vi "NotifyWithDataOverride.vi"(8 "error in (no error)":errorcluster, 11 "TCP Com in":refnum<class "TCP Com.lvclass">) -> (0 "error out":errorcluster, 2 "Data out":refnum<class "Data.lvclass">, 3 "TCP Com out":refnum<class "TCP Com.lvclass">)   [LabVIEW 2023, in "TCP Com.lvclass"]
uses:
  TCP Com.lvclass
  C:/Users/santharu.subramanian/Desktop/LOA New/Documents/LV New Assignments/Sender-Receiver/Classes/Communication/Communication.lvclass
  Data/Data.lvclass
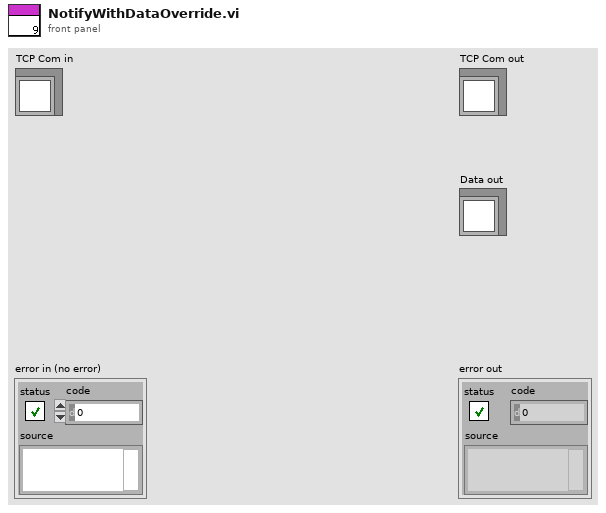
[diagram p1: front panel]
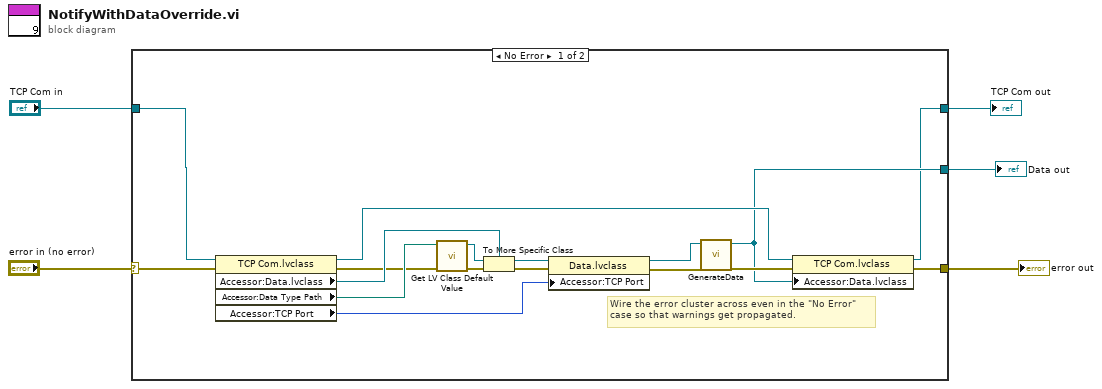
[diagram p0: block diagram]
diagram:
  n1 = case shown="No Error" "error in (no error)" {
    selector: "error in (no error)" -> [w7 w24]
    tunnel: [w6 w24] -> w4
    tunnel: [w8 w23] -> w2
    tunnel: "TCP Com in" -> [w10 w23]
    tunnel: [w9 _] -> w1
    frame No Error {
      # "Wire the error cluster across even in the \"No Error\"\ncase so that warnings get propagated."
      n2 = property class="TCP Com.lvclass"(reference=w10, error in=w7) -> (reference out=w16:refnum<class "TCP Com.lvclass">, error out=w17:errorcluster, "Accessor:Data.lvclass"=w18:refnum<class "Data.lvclass">, "Accessor:Data Type Path"=w19:path, "Accessor:TCP Port"=w11:u16)
      n3 = call <vilib>:"Get LV Class Default Value.vi"("error in (no error)"=w17, "class path"=w19) -> ("error out"=w22:errorcluster, "object"=w21:refnum<class>)  [unwired: 8 in]
      n4 = To More Specific Class(target class=w18, reference=w21, error in=w22) -> (specific class reference=w20:refnum<class "Data.lvclass">, error out=w13:errorcluster)
      n5 = property class="Data.lvclass"(reference=w20, error in=w13, "Accessor:TCP Port"=w11) -> (reference out=w14:refnum<class "Data.lvclass">, error out=w12:errorcluster)
      n6 = call-dynamic "GenerateData.vi"("error in (no error)"=w12, "Data in"=w14) -> ("error out"=w15:errorcluster, "Data out"=w9:refnum<class "Data.lvclass">)  [unwired: 8 in]
      n7 = property class="TCP Com.lvclass"(reference=w16, error in=w15, "Accessor:Data.lvclass"=w9) -> (reference out=w8:refnum<class "TCP Com.lvclass">, error out=w6:errorcluster)
    }
    frame Error {
    }
  }
  "error out" <- w4
  "TCP Com out" <- w2
  "Data out" <- w1
